vi "Loader Post-Build Action.vi"(5 "Files Generated by Build":path[](array[path]), 6 "Top Level/Always Included VIs":path[](array[path]), 7 "Destination Path":path, 8 "error in (no error)":errorcluster, 9 "Target Name":string, 10 "Build Specification Name":string, 11 "Project Path":path) -> (0 "error out":errorcluster)   [LabVIEW 2021, in "CIF Build Actions.lvlib"]
uses:
  CIFConfigurationFile/typedef/Location Type.ctl
  CIFConfigurationFile/CIF Configuration File Location.vi
  <vilib>/CIF Foundation/CIF Utilities/File/File/Prune to Directory.vi
  <vilib>/Utility/error.llb/Clear Errors.vi
  <vilib>/Utility/libraryn.llb/Check if File or Folder Exists.vi
  CIF Build Actions.lvlib
  <vilib>/CIF Foundation/CIF Utilities/File/File_CIF_U.lvlib
  CIFConfigurationFile/CIF Configuration File.lvlib
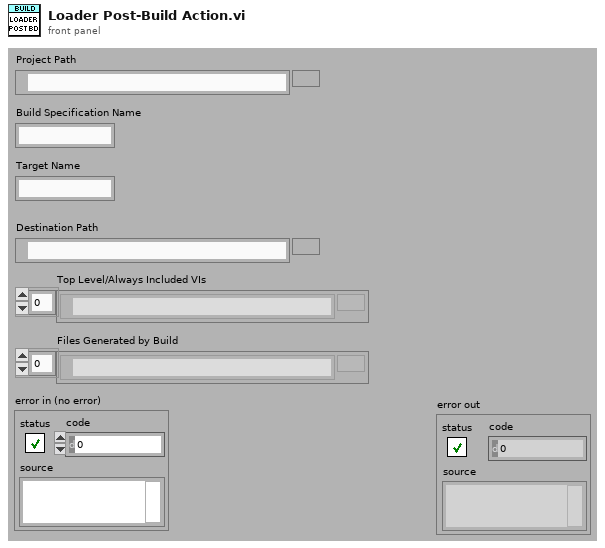
[diagram p1: front panel]
types:
  T1 = typedef "CIF Configuration File.lvlib/Location Type.ctl" = enum16{"Config File", "Manager", "Protos", "Plugins", "UI Plugins", "Logs", "Orchestrations", "Loaders"}
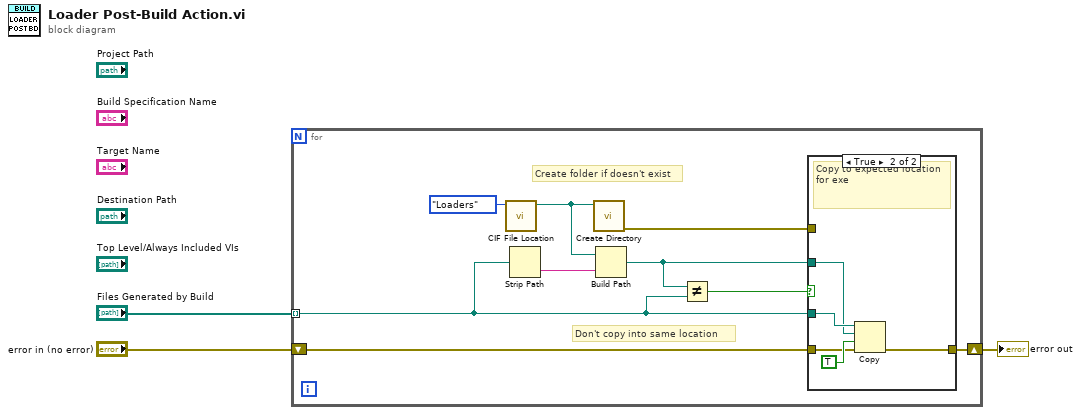
[diagram p0: block diagram]
diagram:
  n1 = for {
    tunnel: "Files Generated by Build" -> [w8] mode=indexing
    shift-right: [w12] -> w1
    shift-left: "error in (no error)" -> [w7]
    # "Create folder if doesn't exist"
    # "Don't copy into same location"
    n2 = call "CIF File Location.vi"("LocationType"=Location_Type."Loaders") -> ("Location"=w4:path)  [unwired: 10 in]
    n3 = Strip Path(path=w8) -> (name=w9:string)  [unwired: 1 out]
    n4 = call <vilib>:"Create Directory.vi"("Path In"=w4) -> ("error out"=w10:errorcluster)  [unwired: 9 in, 1 out]
    n5 = Build Path(base path=w4, name or relative path=w9) -> (appended path=w11:path)
    n6 = Not Equal?(x=w11, y=w8) -> (x != y?=w6:bool)
    n7 = case shown="True" w6 {
      tunnel: w8 -> [_ w18]
      tunnel: w11 -> [_ w17]
      tunnel: w7 -> [w13 w15]
      tunnel: [w13 w14] -> w12
      tunnel: w10 -> [_ _]
      frame False {
        # "PPL not found, could provide error"
      }
      frame True {
        # "Copy to expected location for exe"
        n8 = Copy(8:w15, 9:TRUE ("overwrite (F)"), 10:w17, 11:w18) -> (0:w14:errorcluster)  [unwired: 1 in, 2 out]
      }
    }
  }
  "error out" <- w1
